vi "Node - Config Reader.vi"(8 "error in (no error)":errorcluster, 11 "Node Data In":T1) -> (0 "error out":errorcluster, 3 "Node Data Out":T1)   [LabVIEW 2016, in "PXImc Router.lvlib"]
uses:
  PXImc Router.lvlib
  Controls/Node Data.ctl
  Controls/Node/Node - PXImc Parameters.ctl
  Controls/Node/Node - Writer Data.ctl
  Controls/Node/Node Ch Properties.ctl
  Controls/Data Type.ctl
  Controls/Node/Node - Readers Data.ctl
  Controls/Node/Node - Reader Data.ctl
  <vilib>/NI Veristand/VeriStand Data/Byte Buffer/Byte Buffer.lvclass/Byte Buffer.ctl
  <vilib>/NI Veristand/VeriStand Data/Byte Buffer/Byte Buffer.Get Buffer Pointer.vi
  <vilib>/NI Veristand/VeriStand Data/Byte Buffer/Byte Buffer.Get Buffer Size.vi
  <vilib>/NI Veristand/VeriStand Data/Memory Management/Memory Management.MoveByteBlock (Pointer).vi
  <vilib>/NI Veristand/VeriStand Data/Pointer Operations/Pointer.New.vi
  <vilib>/NI Veristand/VeriStand Data/Pointer Operations/Pointer.Dispose.vi
  <vilib>/NI Veristand/VeriStand Data/Byte Buffer/Byte Buffer.Set Buffer Pointer.vi
  <vilib>/NI Veristand/VeriStand Data/Byte Buffer/Byte Buffer.Set Buffer Size.vi
  <vilib>/NI Veristand/VeriStand Data/Memory Management/Memory Management.Handle Return.vi
  <vilib>/NI Veristand/VeriStand Data/Byte Buffer/Byte Buffer.lvclass
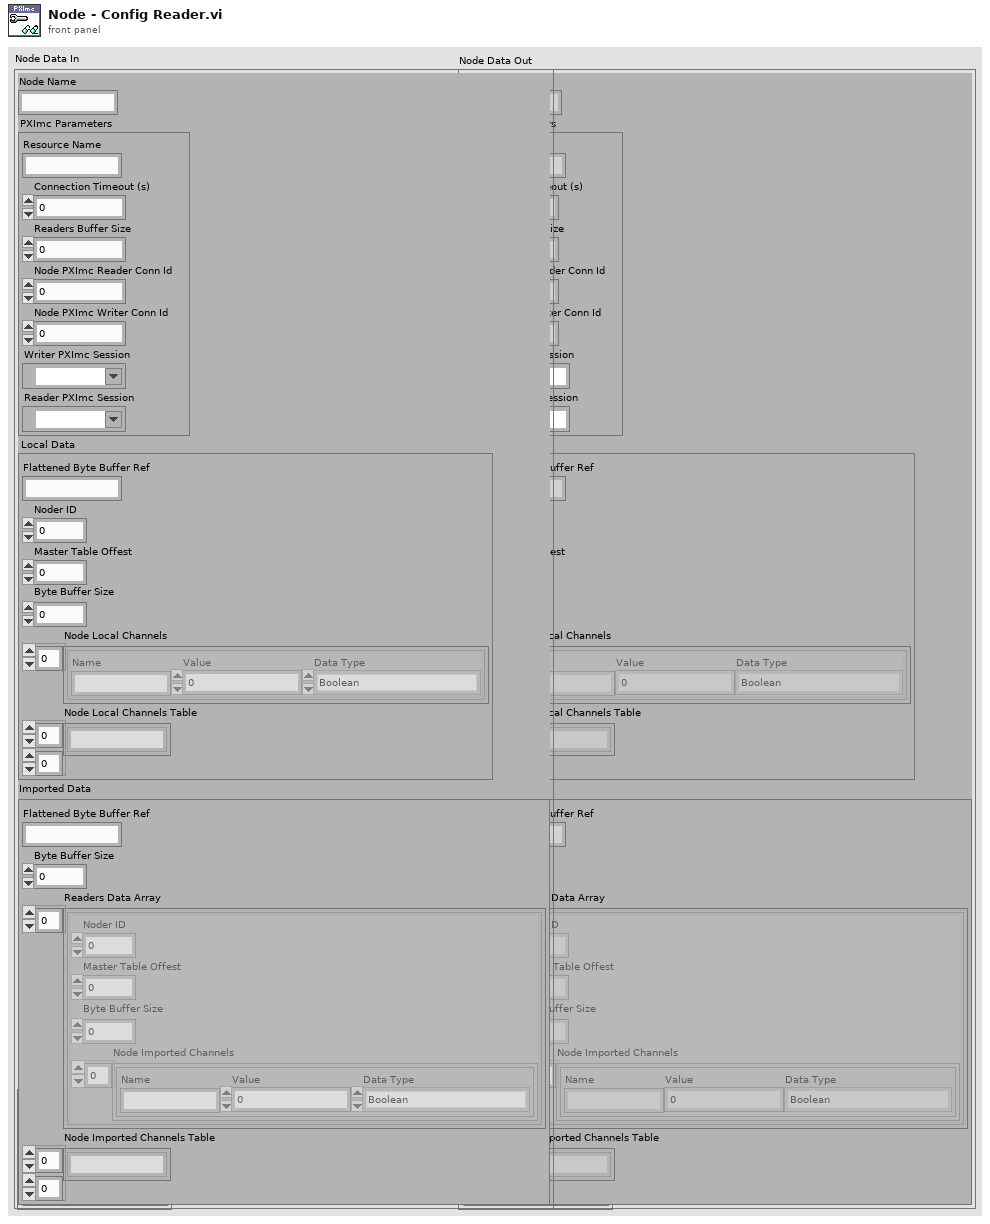
[diagram p1: front panel]
types:
  T1 = typedef "PXImc Router.lvlib/Node Data.ctl" = cluster{"Node Name":string, "PXImc Parameters":T2, "Local Data":T3, "Imported Data":T6}
  T2 = typedef "PXImc Router.lvlib/Node - PXImc Parameters.ctl" = cluster{"Resource Name":string, "Connection Timeout (s)":dbl, "Readers Buffer Size":u64, "Node PXImc Reader Conn Id":u16, "Node PXImc Writer Conn Id":u16, "Writer PXImc Session":refnum<k21>, "Reader PXImc Session":refnum<k21>}
  T3 = typedef "PXImc Router.lvlib/Node - Writer Data.ctl" = cluster{"Flattened Byte Buffer Ref":string, "Noder ID":u32, "Master Table Offest":u32, "Byte Buffer Size":u32, "Node Local Channels":T4[], "Node Local Channels Table":string[][]}
  T4 = typedef "PXImc Router.lvlib/Node Ch Properties.ctl" = cluster{"Name":string, "Value":dbl, "Data Type":T5}
  T5 = typedef "PXImc Router.lvlib/Data Type.ctl" = enum16{"Boolean", "SGL", "DBL", "I8", "I16", "I32", "I64", "U8", "U16", "U32", "U64"}
  T6 = typedef "PXImc Router.lvlib/Node - Readers Data.ctl" = cluster{"Flattened Byte Buffer Ref":string, "Byte Buffer Size":u64, "Readers Data Array":T7[], "Node Imported Channels Table":string[][]}
  T7 = typedef "PXImc Router.lvlib/Node - Reader Data.ctl" = cluster{"Noder ID":u32, "Master Table Offest":u32, "Byte Buffer Size":u64, "Node Imported Channels":T4[]}
  T8 = typedef "PXImc Router.lvlib/Node - Buffer Offsets - Indexes.ctl" = cluster{"Buffer Offsets":u64, "Indexes":i32}
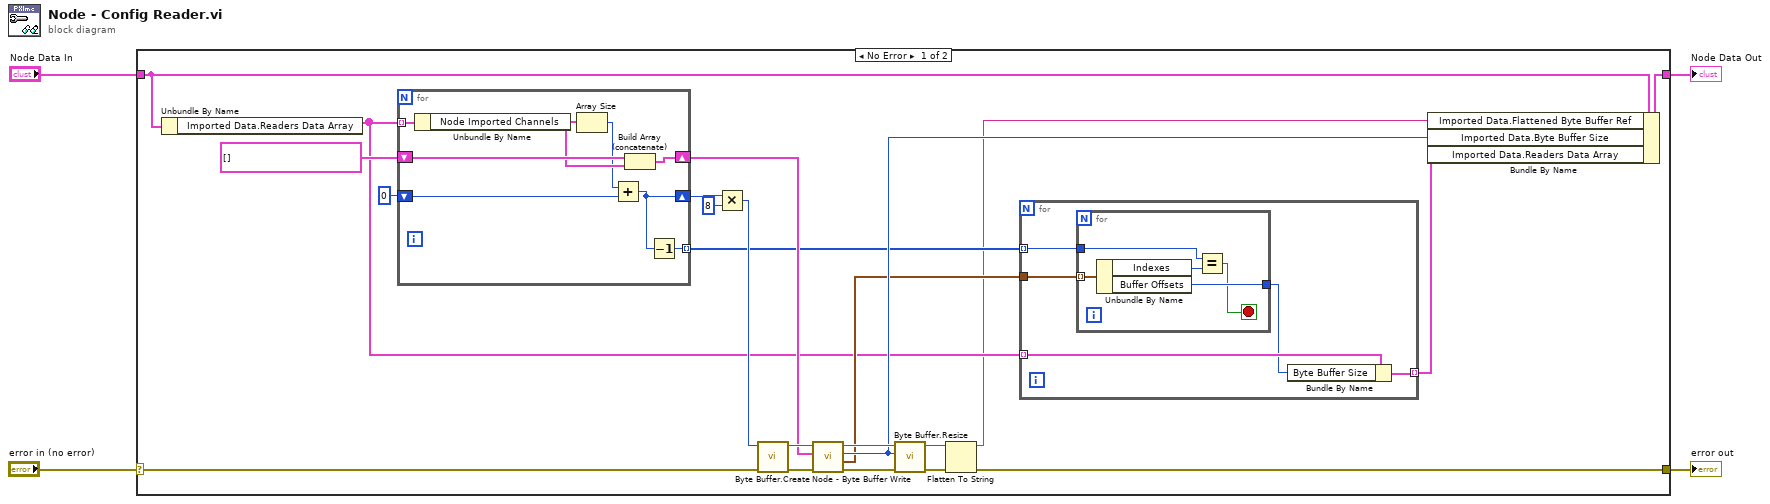
[diagram p0: block diagram]
diagram:
  n1 = case shown="No Error" "error in (no error)" {
    selector: "error in (no error)" -> [w20 w46]
    tunnel: [w26 w45] -> w4
    tunnel: [w6 w46] -> w3
    tunnel: "Node Data In" -> [w11 w45]
    frame No Error {
      n2 = Unbundle By Name(w11) -> ("Imported Data.Readers Data Array"=w10:T7[])
      n3 = for {
        tunnel: w10 -> [w44] mode=indexing
        shift-right: [w38] -> w15
        shift-left: 0 ("x*y") -> [w43]
        shift-right: [w40] -> w17
        shift-left: T4[] [] ("Node Local Channels") -> [w42]
        tunnel: [w37] -> w13 mode=indexing
        n4 = Unbundle By Name(w44) -> ("Node Imported Channels"=w41:T4[])
        n5 = Array Size(array=w41) -> (size(s)=w39:i32)
        n6 = Add(x=w39, y=w43) -> (x+y=w38:i32)
        n7 = Build Array (concatenate)(w42, w41) -> (w40:T4[])
        n8 = Decrement(x=w38) -> (x-1=w37:i32)
      }
      n9 = Multiply(x=w15, y=8) -> (x*y=w19:i32)
      n10 = call <vilib>:"Byte Buffer.Create.vi"("error in (no error)"=w20, "size"=w19) -> ("error out"=w21:errorcluster, "Byte Buffer"=w18:refnum<class "Byte Buffer.lvclass">)  [unwired: 8 in]
      n11 = call "Node - Byte Buffer Write.vi"("error in (no error)"=w21, "Node Local Channels"=w17, "Byte Buffer In"=w18) -> ("error out"=w22:errorcluster, "Buffer Offsets - Indexes Out"=w12:T8[], "Buffer Offset Out"=w16:u64, "Byte Buffer Out"=w23:refnum<class "Byte Buffer.lvclass">)  [unwired: 5 in]
      n12 = call <vilib>:"Byte Buffer.Resize.vi"("error in (no error)"=w22, "new size"=w16, "Byte Buffer in"=w23) -> ("error out"=w7:errorcluster, "Byte Buffer out"=w8:refnum<class "Byte Buffer.lvclass">)  [unwired: 7 in]
      n13 = Flatten To String(anything=w8, error in (no error)=w7) -> (data string=w5:string, error out=w6:errorcluster)  [unwired: 2 in, 1 out]
      n14 = for {
        tunnel: w13 -> [w30] mode=indexing
        tunnel: w12 -> [w31]
        tunnel: w10 -> [w29] mode=indexing
        tunnel: [w27] -> w9 mode=indexing
        n15 = for {
          tunnel: w31 -> [w36] mode=indexing
          tunnel: w30 -> [w34]
          tunnel: [w33] -> w28
          stop <- w32 stop-if-true
          n16 = Unbundle By Name(w36) -> ("Indexes"=w35:i32, "Buffer Offsets"=w33:u64)
          n17 = Equal?(x=w34, y=w35) -> (x = y?=w32:bool)
        }
        n18 = Bundle By Name(cluster=w29, "Byte Buffer Size"=w28) -> (w27:T7)
      }
      n19 = Bundle By Name(cluster=w11, "Imported Data.Flattened Byte Buffer Ref"=w5, "Imported Data.Byte Buffer Size"=w16, "Imported Data.Readers Data Array"=w9) -> (w26:T1)
    }
    frame Error {
    }
  }
  "error out" <- w3
  "Node Data Out" <- w4
